vi "Offset and Multiplier to Array.vi"(1 "Size":i32, 2 "Offset and Multiplier":T1) -> (0 "Array":dbl[](array[numeric]))   [LabVIEW 2016, in "graph_utilities.lvclass"]
doc: "Calculate an Array for the given Offset and Multiplier"
uses:
  graph_utilities.lvclass
  <vilib>/Utility/miscctls.llb/LVOffsetAndMultiplierTypeDef.ctl
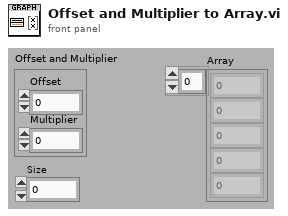
[diagram p1: front panel]
types:
  T1 = typedef "LVOffsetAndMultiplierTypeDef.ctl" = cluster{"Offset":dbl, "Multiplier":dbl}
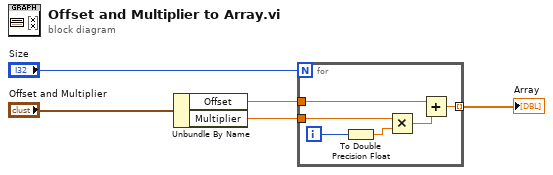
[diagram p0: block diagram]
diagram:
  n1 = Unbundle By Name("Offset and Multiplier") -> ("Offset"=w1:dbl, "Multiplier"=w2:dbl)
  n2 = for {
    N: "Size" -> [_]
    tunnel: w1 -> [w9]
    tunnel: w2 -> [w11]
    tunnel: [w8] -> w5 mode=indexing
    i -> [w10]
    n3 = To Double Precision Float(number=w10) -> (double precision float=w7:dbl)
    n4 = Multiply(x=w11, y=w7) -> (x*y=w6:dbl)
    n5 = Add(x=w9, y=w6) -> (x+y=w8:dbl)
  }
  "Array" <- w5
